vi "worksheet set header opt.vi"(8 "error in (no error)":errorcluster, 9 "options":T1, 10 "string":string, 11 "worksheet":u32) -> (0 "error out":errorcluster, 1 "options out":T1, 3 "function return":u32(ring))   [LabVIEW 8.6]
doc: "lxw_error worksheet_set_header_opt(lxw_worksheet worksheet, const char *string, lxw_header_footer_options *options);"
uses:
  pending_lvxlsxwriter/xlsxwriter.dll
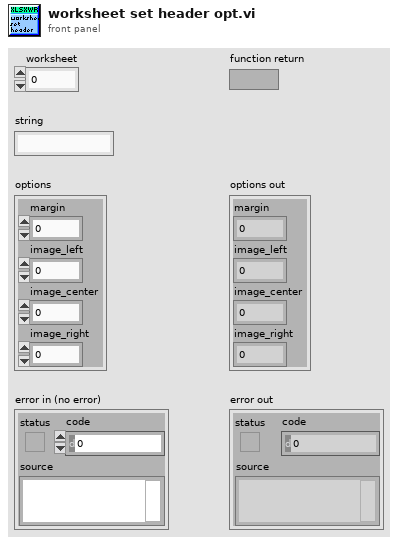
[diagram p1: front panel]
types:
  T1 = cluster{"margin":dbl, "image_left":u32, "image_center":u32, "image_right":u32}
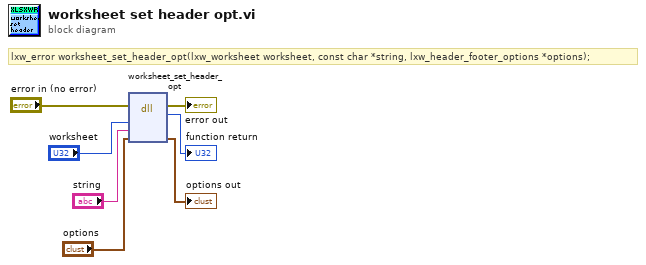
[diagram p0: block diagram]
diagram:
  # "lxw_error worksheet_set_header_opt(lxw_worksheet worksheet, const char *string, lxw_header_footer_options *options);"
  n1 = dll-call lib="C:/Users/WDAGUtilityAccount/Desktop/pending_lvxlsxwriter/xlsxwriter.*" fn="worksheet_set_header_opt"(error in="error in (no error)", "worksheet"="worksheet", "string"="string", "options"="options") -> (error out=→"error out":errorcluster, →"function return":u32, "options"=→"options out":T1)  [unwired: 4 in, 1 out]
